vi "Function Generator & Spectrum Analyzer.vi"() -> ()   [LabVIEW 2020]
uses:
  <vilib>/measure/maspectr.llb/FFT Power Spectrum and PSD for 1 Chan.vi
  <vilib>/measure/NI_MABase.lvlib
  <vilib>/measure/NI_MAPro.lvlib
panel:
  in  "Stop":bool
  in  "Noise":dbl(knob) scale=0.0..10.0
  in  "Offset":dbl(knob) scale=0.0..10.0
  in  "Wave Selector":T1(ring)
  in  "Phase":dbl(knob) scale=0.0..10.0
  in  "Amplitude":dbl(knob) scale=0.0..10.0
  in  "Frequency":dbl(knob) scale=0.0..10.0
  out "Frequency Domain":cluster{"f0":dbl, "df":dbl, "magnitude":dbl[]}(graph)
  out "Time Domain":waveform(dbl)(graph)
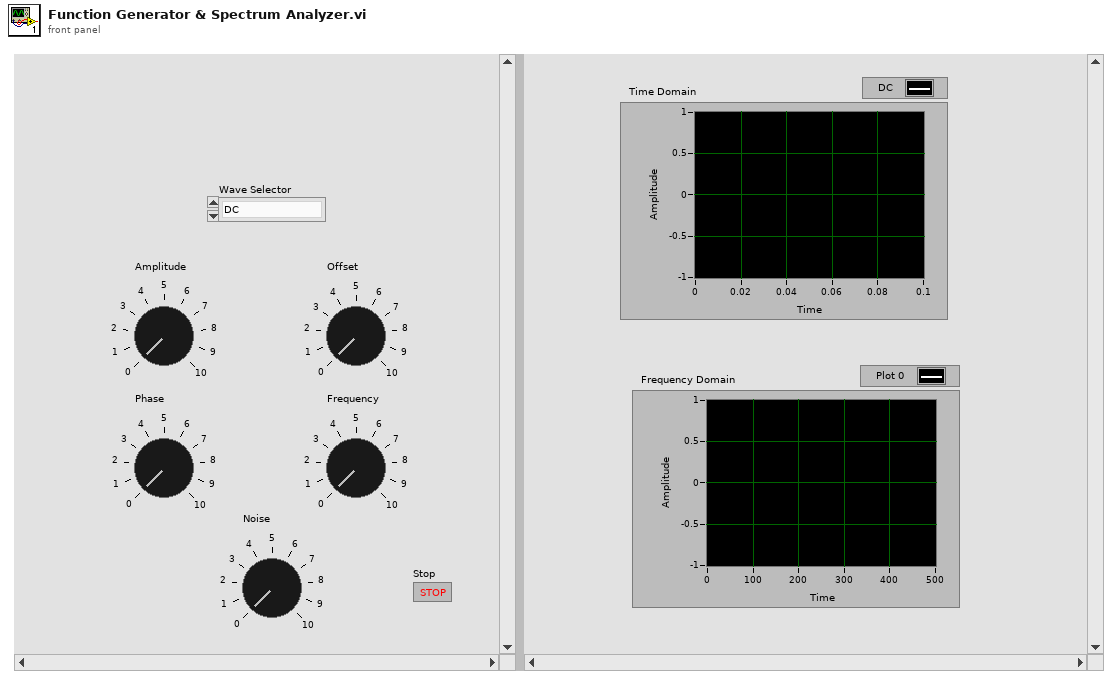
[diagram p1: front panel]
types:
  T1 = enum16{"DC", "Triangle", "Sawtooth", "Square", "Sine"}
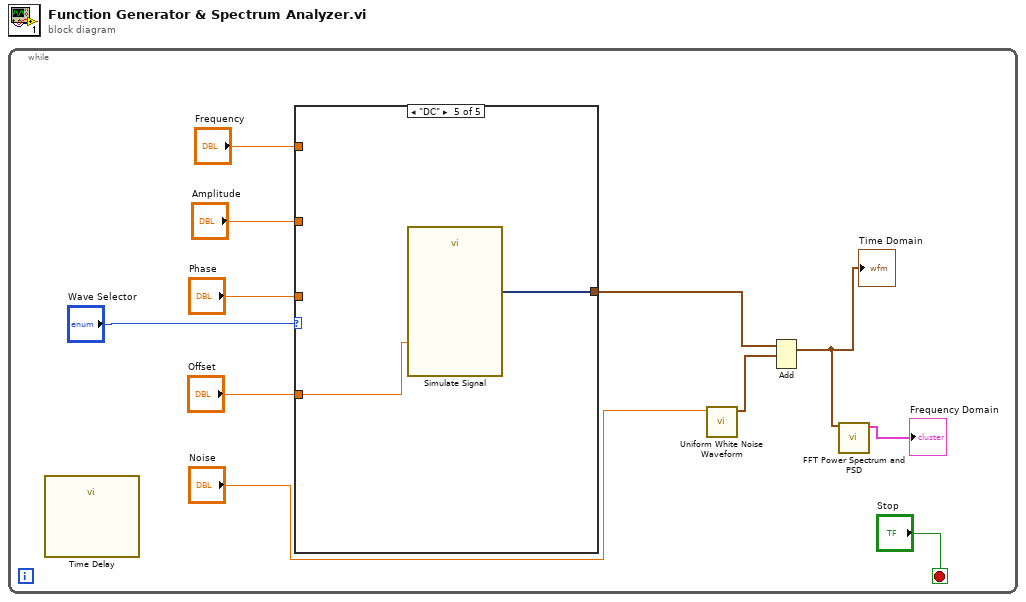
[diagram p0: block diagram]
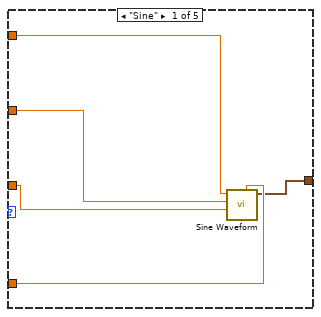
[diagram p2: hidden frame]
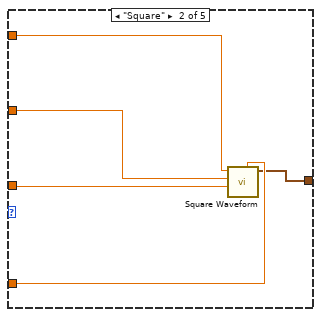
[diagram p3: hidden frame]
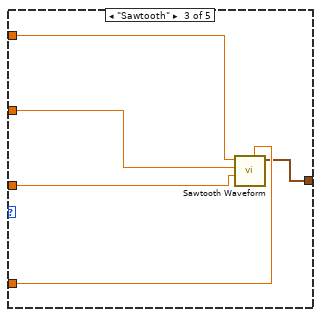
[diagram p4: hidden frame]
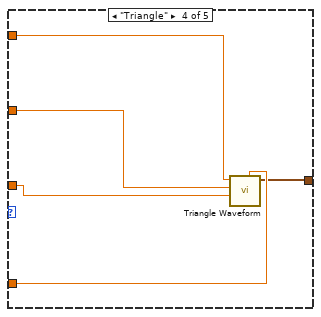
[diagram p5: hidden frame]
diagram:
  n1 = while {
    stop <- "Stop" stop-if-true
    n2 = call "Time Delay"() -> ()  [unwired: 11 in, 1 out]
    n3 = case shown="\"DC\"" "Wave Selector" {
      tunnel: "Frequency" -> [w16 w21 w26 w31 _]
      tunnel: "Amplitude" -> [w15 w20 w25 w30 _]
      tunnel: "Phase" -> [w14 w19 w24 w29 _]
      tunnel: "Offset" -> [w13 w18 w23 w28 w33]
      tunnel: [w12 w17 w22 w27 w32] -> w6
      frame "Sine" {
        n4 = call <vilib>:"Sine Waveform.vi"("offset"=w13, "phase"=w14, "amplitude"=w15, "frequency"=w16) -> ("signal out"=w12:waveform(dbl))  [unwired: 6 in, 1 out]
      }
      frame "Square" {
        n5 = call <vilib>:"Square Waveform.vi"("offset"=w18, "phase"=w19, "amplitude"=w20, "frequency"=w21) -> ("signal out"=w17:waveform(dbl))  [unwired: 6 in, 1 out]
      }
      frame "Sawtooth" {
        n6 = call <vilib>:"Sawtooth Waveform.vi"("offset"=w23, "phase"=w24, "amplitude"=w25, "frequency"=w26) -> ("signal out"=w22:waveform(dbl))  [unwired: 6 in, 1 out]
      }
      frame "Triangle" {
        n7 = call <vilib>:"Triangle Waveform.vi"("offset"=w28, "phase"=w29, "amplitude"=w30, "frequency"=w31) -> ("signal out"=w27:waveform(dbl))  [unwired: 6 in, 1 out]
      }
      frame "DC" {
        n8 = call "Simulate Signal"("Offset"=w33) -> ("DC"=w32:dynamicdata)  [unwired: 13 in, 1 out]
      }
    }
    n9 = call <vilib>:"Uniform White Noise Waveform.vi"("amplitude"="Noise") -> ("signal out"=w3:waveform(dbl))  [unwired: 9 in, 1 out]
    n10 = Add(1:w3, 2:w6) -> (0:w2:waveform(dbl))  [unwired: 1 in, 1 out]
    "Time Domain" <- w2
    n11 = call-poly <vilib>:"FFT Power Spectrum and PSD.vi"("time signal"=w2) -> ("Power Spectrum / PSD"=→"Frequency Domain":cluster{"f0":dbl, "df":dbl, "magnitude":dbl[]})  [unwired: 7 in, 3 out]
  }
